vi "fgt set pressure Unit.vi"(8 "error in (no error)":errorcluster, 10 "unit":T1, 11 "presureIndex":u32) -> (0 "error out":errorcluster)   [LabVIEW 2020, in "fgt_SDK.lvlib"]
doc: "Set pressure unit on selected pressure device, default value is \"mbar\". If type is invalid an error is returned.\nEvery pressure read value and sent command will then use this unit.\nExample of type: \"mbar\", \"millibar\", \"kPa\" ..."
uses:
  fgt_SDK.lvlib
  TypeDefs/fgt_PRESSURE_UNIT.ctl
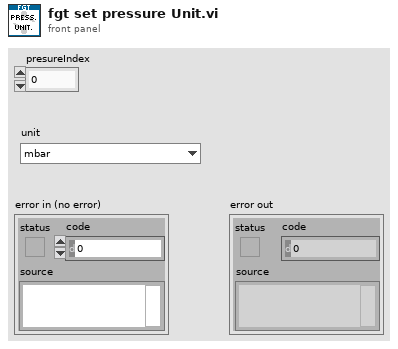
[diagram p1: front panel]
types:
  T1 = typedef "fgt_SDK.lvlib/fgt_PRESSURE_UNIT.ctl" = enum16{"mbar", "kPa", "PSI"}
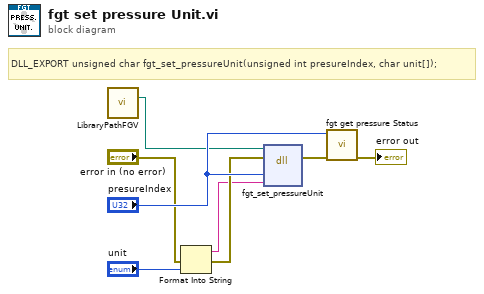
[diagram p0: block diagram]
diagram:
  # "DLL_EXPORT unsigned char fgt_set_pressureUnit(unsigned int presureIndex, char unit[]);"
  n1 = call "LibraryPathFGV.vi"() -> ("Path Out"=w1:path)  [unwired: 14 in, 1 out]
  n2 = Format Into String(error in="error in (no error)", "unit") -> (resulting string=w2:string, error out=w3:errorcluster)  [unwired: 2 in]
  n3 = dll-call lib="C:/Workspace/fgt-SDK/LabVIEW/dlls/fgt_SDK_*.*" fn="fgt_set_pressureUnit"(path in=w1, error in=w3, "presureIndex"="presureIndex", "unit"=w2) -> (error out=w8:errorcluster)  [unwired: 4 in, 1 out]
  n4 = call "fgt get pressure Status.vi"("error in (no error)"=w8, "pressureIndex"="presureIndex") -> ("error out"=→"error out":errorcluster)  [unwired: 9 in]
